vi "Set Limits.vi"(5 "- Limit Value (-5)":dbl=-5.0, 7 "+ Limit Value (5)":dbl=5.0, 8 "error in":errorcluster, 10 "Limit Value Type (0: Volts)":i32(ring) items=["Volts", "Current"], 11 "COM Port":string="COM3") -> (0 "error out":errorcluster)   [LabVIEW 2015]
uses:
  <instrlib>/Fluke 5080/Fluke 5080.lvlib
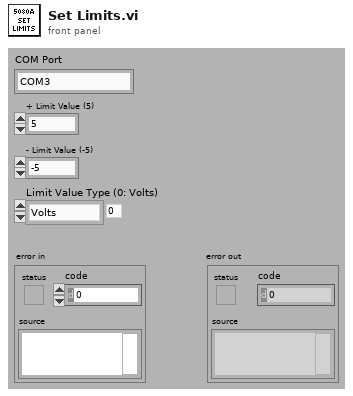
[diagram p1: front panel]
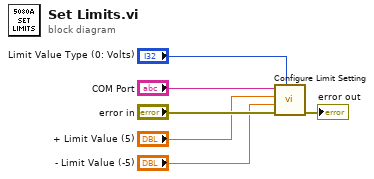
[diagram p0: block diagram]
diagram:
  n1 = call <instrlib>:"Configure Limit Setting.vi"("Limit Value Type (0: Volts)"="Limit Value Type (0: Volts)", "error in (no error)"="error in", "- Limit Value (-5)"="- Limit Value (-5)", "+ Limit Value (5)"="+ Limit Value (5)", "VISA resource name"="COM Port") -> ("error out"=→"error out":errorcluster)  [unwired: 6 out]
